vi "Untitled 1.vi"   [LabVIEW 2011]
types:
  T1 = typedef "LVAllMonitorsDisplayTypeDef.ctl" = cluster{"Bounds":cluster{"Left":i16, "Top":i16, "Right":i16, "Bottom":i16}, "Depth":i16}[]
  T2 = cluster{"Disp.AllMonitors[0]":cluster{"Bounds":cluster{"Left":i16, "Top":i16, "Right":i16, "Bottom":i16}, "Depth":i16}, "Disp.AllMonitors[1]":cluster{"Bounds":cluster{"Left":i16, "Top":i16, "Right":i16, "Bottom":i16}, "Depth":i16}, "Disp.AllMonitors[2]":cluster{"Bounds":cluster{"Left":i16, "Top":i16, "Right":i16, "Bottom":i16}, "Depth":i16}, "Disp.AllMonitors[3]":cluster{"Bounds":cluster{"Left":i16, "Top":i16, "Right":i16, "Bottom":i16}, "Depth":i16}, "Disp.AllMonitors[4]":cluster{"Bounds":cluster{"Left":i16, "Top":i16, "Right":i16, "Bottom":i16}, "Depth":i16}, "Disp.AllMonitors[5]":cluster{"Bounds":cluster{"Left":i16, "Top":i16, "Right":i16, "Bottom":i16}, "Depth":i16}, "Disp.AllMonitors[6]":cluster{"Bounds":cluster{"Left":i16, "Top":i16, "Right":i16, "Bottom":i16}, "Depth":i16}, "Disp.AllMonitors[7]":cluster{"Bounds":cluster{"Left":i16, "Top":i16, "Right":i16, "Bottom":i16}, "Depth":i16}, "Disp.AllMonitors[8]":cluster{"Bounds":cluster{"Left":i16, "Top":i16, "Right":i16, "Bottom":i16}, "Depth":i16}}
  T3 = cluster{"Left":i16, "Top":i16, "Right":i16, "Bottom":i16}
  T4 = typedef "LVPointTypeDef.ctl" = cluster{"Horizontal":i16, "Vertical":i16}
  T5 = cluster{"Left":bool, "Top":bool, "Right":bool, "Bottom":bool}
  T6 = typedef "LVRectTypeDef.ctl" = cluster{"left":i16, "top":i16, "right":i16, "bottom":i16}
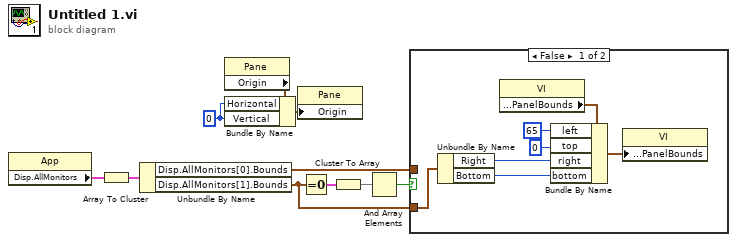
[diagram p0: block diagram]
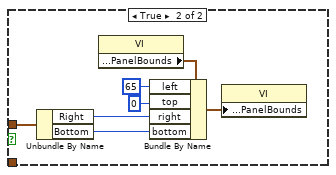
[diagram p2: hidden frame]
diagram:
  w4 = i16 0 ("Vertical")
  n1 = property class="App"() -> ("Disp.AllMonitors"=w1:T1)  [unwired: 2 in, 2 out]
  n2 = Array To Cluster(array=w1) -> (cluster=w5:T2)
  n3 = Unbundle By Name(w5) -> ("Disp.AllMonitors[0].Bounds"=w9:T3, "Disp.AllMonitors[1].Bounds"=w10:T3)
  n4 = property on="Property Node" class="Pane"() -> ("Origin"=w3:T4)  [unwired: 2 in, 2 out]
  n5 = Bundle By Name(cluster=w3, "Horizontal"=w4, "Vertical"=w4) -> (w2:T4)
  n6 = property on="Property Node" class="Pane"("Origin"=w2) -> ()  [unwired: 2 in, 2 out]
  n7 = Equal To 0?(x=w10) -> (x = 0?=w6:T5)
  n8 = Cluster To Array(cluster=w6) -> (array=w7:bool[])
  n9 = And Array Elements(Boolean array=w7) -> (logical AND=w8:bool)
  n10 = case shown="False" w8 {
    tunnel: w9 -> [_ w20]
    tunnel: w10 -> [w11 _]
    frame False {
      n11 = Unbundle By Name(w11) -> ("Right"=w13:i16, "Bottom"=w12:i16)
      n12 = property class="VI"() -> ("Front Panel.PanelBounds"=w14:T6)  [unwired: 2 in, 2 out]
      n13 = Bundle By Name(cluster=w14, "left"=i16 65, "top"=i16 0, "right"=w13, "bottom"=w12) -> (w15:T6)
      n14 = property class="VI"("Front Panel.PanelBounds"=w15) -> ()  [unwired: 2 in, 2 out]
    }
    frame True {
      n15 = Unbundle By Name(w20) -> ("Right"=w19:i16, "Bottom"=w18:i16)
      n16 = property class="VI"() -> ("Front Panel.PanelBounds"=w21:T6)  [unwired: 2 in, 2 out]
      n17 = Bundle By Name(cluster=w21, "left"=i16 65, "top"=i16 0, "right"=w19, "bottom"=w18) -> (w22:T6)
      n18 = property class="VI"("Front Panel.PanelBounds"=w22) -> ()  [unwired: 2 in, 2 out]
    }
  }
